vi "Get MethodsCalled.vi"(11 "MockListImp":refnum<class "ListImp_RefSpy.lvclass">) -> (2 "MethodsCalled":string[](array[string]), 3 "MockListImp out":refnum<class "ListImp_RefSpy.lvclass">)   [LabVIEW 2013, in "ListImp_RefSpy.lvclass"]
uses:
  ListImp_RefSpy.lvclass
  RefnumGlobal.vi
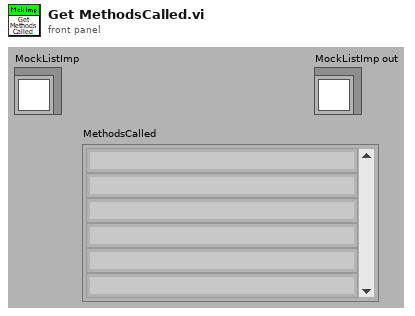
[diagram p1: front panel]
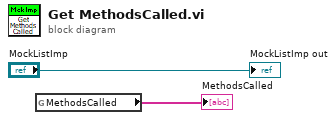
[diagram p0: block diagram]
diagram:
  n1 = global read "RefnumGlobal.vi" "MethodsCalled"() -> (→"MethodsCalled":string[])
  "MockListImp out" <- "MockListImp"
